vi "set_controls_enabled_state.vi"(8 "error in (no error)":errorcluster, 9 "status":T1(ring), 10 "control references":refnum<vi>[](array[refnum]), 11 "ImagingModeDL090130Frame in":refnum<class "ImagingModeDL090130Frame.lvclass">=refnum) -> (0 "error out":errorcluster, 3 "ImagingModeDL090130Frame out":refnum<class "ImagingModeDL090130Frame.lvclass">)   [LabVIEW 2010, in "ImagingModeDL090130Frame.lvclass"]
uses:
  ImagingModeDL090130Frame.lvclass
  main/labview_source/type_definitions/enumerations/run_mode_enum.ctl
  ImagingModeDL090130Frame.lvclass/ImagingModeDL090130Frame.ctl
  common/classes/GenericComponent/GenericComponent/class_data.vi
  common/classes/ErrorController/ErrorController/class_data.vi
  common/classes/ErrorController/ErrorController/ErrorController.lvclass
  common/classes/GenericComponent/GenericComponent/GenericComponent.lvclass
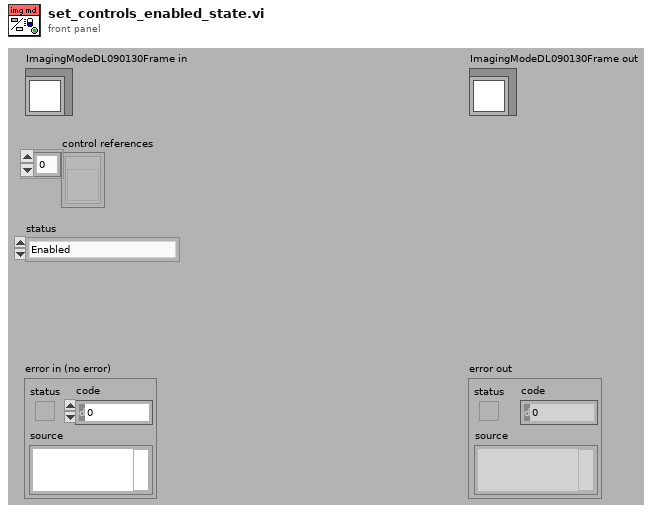
[diagram p1: front panel]
types:
  T1 = enum8{"Enabled", "Disabled", "Disabled and Grayed Out"}
  T2 = typedef "run_mode_enum.ctl" = enum16{"focus mode", "single sweep mode", "experiment mode"}
  T3 = typedef "ImagingModeDL090130Frame.lvclass/control_refs.ctl" = cluster{"resolution controls":cluster{"x pixels":refnum<vi>, "y pixels":refnum<vi>, "ratio x factor":refnum<vi>, "ratio y factor":refnum<vi>, "center(xgalvo,V)":refnum<vi>, "center(ygalvo,V)":refnum<vi>, "amplitude(ygalvo,V)":refnum<vi>, "amplitude(xgalvo,V)":refnum<vi>, "xy galvo view?":refnum<vi>}, "speed controls":cluster{"pixel dwell time":refnum<vi>, "line scan time":refnum<vi>, "frame rate":refnum<vi>, "keep constant":refnum<vi>}, "number of frames controls":cluster{"# of frames":refnum<vi>, "duration":refnum<vi>, "# of repetitions":refnum<vi>}, "current value indicators":cluster{"frame #":refnum<vi>, "repetition #":refnum<vi>, "offset":refnum<vi>}, "step controls":cluster{"step size":refnum<vi>, "return to origin?":refnum<vi>, "translation mode":refnum<vi>, "XIntensityCompensation":refnum<vi>}, "defineButton":refnum<vi>, "settings enforced?":refnum<vi>, "settings":refnum<vi>}
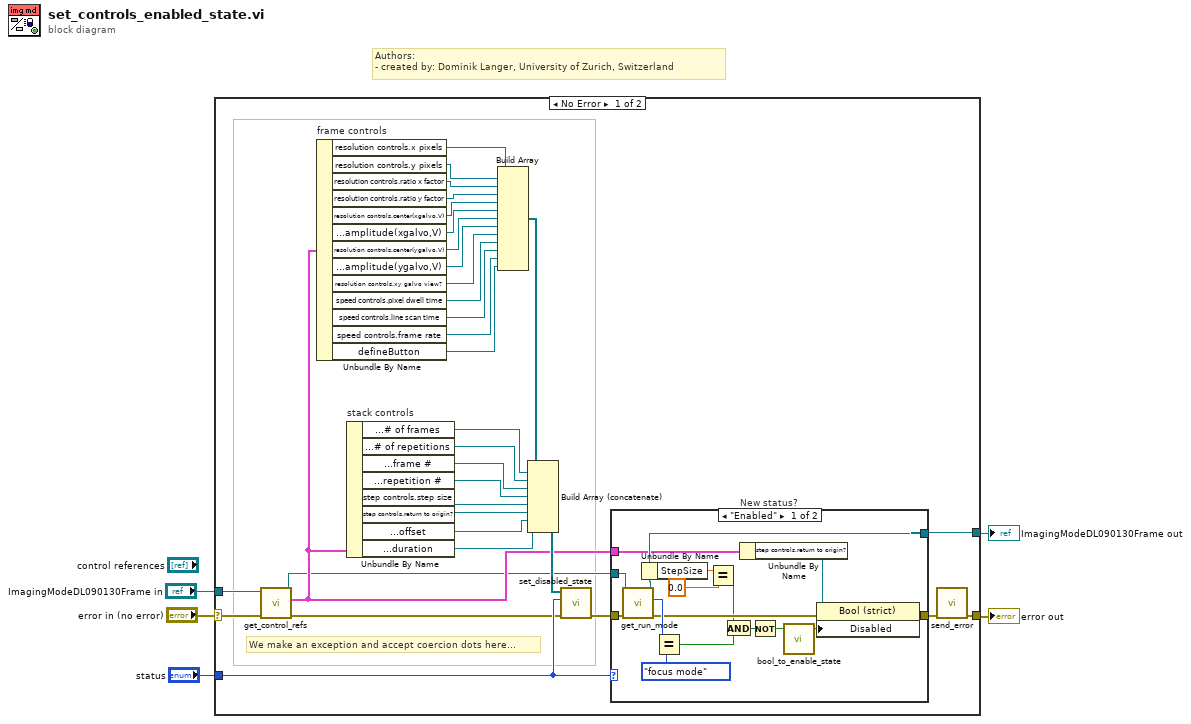
[diagram p0: block diagram]
diagram:
  # "Authors: \n- created by: Dominik Langer, University of Zurich, Switzerland"
  n1 = case shown="No Error" "error in (no error)" {
    selector: "error in (no error)" -> [w19 w58]
    tunnel: [w21 w58] -> w4
    tunnel: [w38 w57] -> w2
    tunnel: "ImagingModeDL090130Frame in" -> [w17 w57]
    tunnel: "status" -> [w24 _]
    frame No Error {
      # "We make an exception and accept coercion dots here..."
      n2 = call-dynamic "get_control_refs.vi"("error in (no error)"=w19, "ImagingModeDL090130Frame in"=w17) -> ("error out"=w18:errorcluster, "control refs"=w16:T3, "ImagingModeDL090130Frame out"=w15:refnum<class "ImagingModeDL090130Frame.lvclass">)  [unwired: 7 in]
      n3 = Unbundle By Name "frame controls"(w16) -> ("resolution controls.x pixels"=w27:refnum<vi>, "resolution controls.y pixels"=w26:refnum<vi>, "resolution controls.ratio x factor"=w28:refnum<vi>, "resolution controls.ratio y factor"=w29:refnum<vi>, "resolution controls.center(xgalvo,V)"=w11:refnum<vi>, "resolution controls.amplitude(xgalvo,V)"=w10:refnum<vi>, "resolution controls.center(ygalvo,V)"=w8:refnum<vi>, "resolution controls.amplitude(ygalvo,V)"=w9:refnum<vi>, "resolution controls.xy galvo view?"=w6:refnum<vi>, "speed controls.pixel dwell time"=w7:refnum<vi>, "speed controls.line scan time"=w12:refnum<vi>, "speed controls.frame rate"=w13:refnum<vi>, "defineButton"=w14:refnum<vi>)
      n4 = Unbundle By Name "stack controls"(w16) -> ("number of frames controls.# of frames"=w37:refnum<vi>, "number of frames controls.# of repetitions"=w36:refnum<vi>, "current value indicators.frame #"=w35:refnum<vi>, "current value indicators.repetition #"=w34:refnum<vi>, "step controls.step size"=w32:refnum<vi>, "step controls.return to origin?"=w30:refnum<vi>, "current value indicators.offset"=w33:refnum<vi>, "number of frames controls.duration"=w31:refnum<vi>)
      n5 = Build Array(w27, w26, w28, w29, w11, w10, w8, w9, w6, w7, w12, w13, w14) -> (w22:refnum<vi>[])
      n6 = Build Array (concatenate)(w22, w37, w36, w35, w34, w32, w30, w33, w31) -> (w23:refnum<vi>[])
      n7 = call "set_disabled_state.vi"("error in"=w18, "status in"=w24, "control references"=w23) -> ("error out"=w25:errorcluster)  [unwired: 8 in]
      n8 = case "New status?" shown="\"Enabled\"" w24 {
        tunnel: w25 -> [w53 w56]
        tunnel: [w54 w56] -> w20
        tunnel: w15 -> [w52 w55]
        tunnel: [w51 w55] -> w38
        tunnel: w16 -> [w47 _]
        frame "Enabled" {
          n9 = call "get_run_mode.vi"("error in (no error)"=w53, "GenericPlugin in"=w52) -> ("error out"=w40:errorcluster, "run mode"=w50:T2, "GenericPlugin out"=w51:refnum<class "ImagingModeDL090130Frame.lvclass">)  [unwired: 5 in, 2 out]
          n10 = Unbundle By Name(w51) -> ("StepSize"=w42:dbl[unit])
          n11 = Equal?(x=w50, y=run_mode_enum."focus mode") -> (x = y?=w48:bool)
          n12 = Equal?(x=w42, y=dbl[unit] 0.0) -> (x = y?=w39:bool)
          n13 = And(x=w39, y=w48) -> (x .and. y?=w45:bool)
          n14 = Unbundle By Name(w47) -> ("step controls.return to origin?"=w46:refnum<vi>)
          n15 = Not(x=w45) -> (.not. x?=w44:bool)
          n16 = call "bool_to_enable_state.vi"("boolean in"=w44) -> ("enabled status out"=w43:T1)  [unwired: 4 in]
          n17 = property class="Bool (strict)"(reference=w46, error in=w40, "Disabled"=w43) -> (error out=w54:errorcluster)  [unwired: 1 out]
        }
        frame "Disabled", Default {
        }
      }
      n18 = call "send_error.vi"("error in (no error)"=w20) -> ("error out"=w21:errorcluster)  [unwired: 10 in]
    }
    frame Error {
    }
  }
  "error out" <- w4
  "ImagingModeDL090130Frame out" <- w2
